vi "DSF Config File to Engine Config Cluster.vi"(8 "error in (no error)":errorcluster, 10 "engine offsets":u64[](array[numeric]), 11 "dsf configuration file path":path) -> (0 "error out":errorcluster, 3 "configuration cluster":T1)   [LabVIEW 2017, in "DSF.Engine.lvlib"]
uses:
  DSF.Engine.lvlib
  Shared/Typedefs/DSF.Shared.Refactor.Typedefs.Framework Configuration.Aggregate.JSON.ctl
  Shared/Typedefs/DSF.Shared.Refactor.Typedefs.Plugin Configuration.Aggregate.JSON.ctl
  Shared/Typedefs/DSF.Shared.Typedefs.Cycle Timing Factors.ctl
  Shared/Typedefs/DSF.Shared.Refactor.Typedefs.Transfer Group Configuration.Aggregate.JSON.ctl
  Shared/Typedefs/DSF.Shared.Refactor.Typedefs.JSON.Transfer Configuration.ctl
  Shared/Typedefs/DSF.Shared.Refactor.Typedefs.JSON.Channel Array Configuration.ctl
  Shared/Typedefs/DSF.Shared.Typedefs.Settings.Configuration.ctl
  DSF Configuration API/1.0.0/Public/Read All Item IDs/Read All Plugin IDs.vi
  DSF Configuration API/1.0.0/Public/Read Item/Read Plugin.vi
  DSF Configuration API/1.0.0/Public/Read Item/Read Settings.vi
  DSF Configuration API/1.0.0/Public/Read Item/Read Group.vi
  DSF Configuration API/1.0.0/Public/Read Item/Read Transfer.vi
  DSF Configuration API/1.0.0/Public/Read Item/Read Channel.vi
  DSF Configuration API/1.0.0/DSF Configuration API.lvlib
  DSF.Shared.lvlib
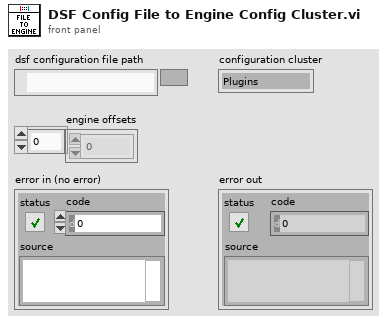
[diagram p1: front panel]
types:
  T1 = typedef "DSF.Shared.lvlib/DSF.Shared.Refactor.Typedefs.Framework Configuration.Aggregate.JSON.ctl" = cluster{"Plugins":T2[]}
  T2 = typedef "DSF.Shared.lvlib/DSF.Shared.Refactor.Typedefs.Plugin Configuration.Aggregate.JSON.ctl" = cluster{"name":string, "class":string, "cycle timing":T3, "Transfer Groups":T4[], "settings":T7[]}
  T3 = typedef "DSF.Shared.lvlib/DSF.Shared.Typedefs.Cycle Timing Factors.ctl" = cluster{"Priority":u64, "Decimation":u64, "Offset":u64}
  T4 = typedef "DSF.Shared.lvlib/DSF.Shared.Refactor.Typedefs.Transfer Group Configuration.Aggregate.JSON.ctl" = cluster{"name":string, "direction":u8, "cycle timing":T3, "Transfers":T5[], "settings":T7[]}
  T5 = typedef "DSF.Shared.lvlib/DSF.Shared.Refactor.Typedefs.JSON.Transfer Configuration.ctl" = cluster{"name":string, "byte order":u8, "channel configurations":T6[], "settings":T7[]}
  T6 = typedef "DSF.Shared.lvlib/DSF.Shared.Refactor.Typedefs.JSON.Channel Array Configuration.ctl" = cluster{"name":string, "data type":u8, "count":u64, "buffer offset":u64, "engine offset":u64, "settings":T7[]}
  T7 = typedef "DSF.Shared.lvlib/DSF.Shared.Typedefs.Settings.Configuration.ctl" = cluster{"key":string, "value":string}
  T8 = typedef "DSF Configuration API.lvlib/DSF Config Data RefNum.ctl" = refnum<k1>
  T9 = typedef "DSF Configuration API.lvlib/DSF Plugin Info.ctl" = cluster{"type":string, "timing":T10, "group ids":string[], "settings id":string}
  T10 = typedef "DSF Configuration API.lvlib/DSF Timing Info.ctl" = cluster{"priority":i32, "decimation":i32, "offset":i32}
  T11 = typedef "DSF Configuration API.lvlib/DSF Settings Info.ctl" = cluster{"key":string, "value":string}[]
  T12 = typedef "DSF Configuration API.lvlib/DSF Group Info.ctl" = cluster{"direction":T13, "timing":T10, "transfer ids":string[], "settings id":string}
  T13 = typedef "DSF Configuration API.lvlib/DSF Direction.ctl" = enum8{"Tx", "Rx"}
  T14 = typedef "DSF Configuration API.lvlib/DSF Transfer Info.ctl" = cluster{"byte order":T15, "channel ids":string[], "settings id":string}
  T15 = typedef "DSF Configuration API.lvlib/DSF Byte Order.ctl" = enum8{"big-endian", "little-endian"}
  T16 = typedef "DSF Configuration API.lvlib/DSF Channel Info.ctl" = cluster{"count":i32, "offset":i32, "data type":T17, "resource path":string, "settings id":string}
  T17 = typedef "DSF Configuration API.lvlib/DSF Data Type.ctl" = enum8{"Bool", "SGL", "DBL", "I8", "I16", "I32", "I64", "U8", "U16", "U32", "U64"}
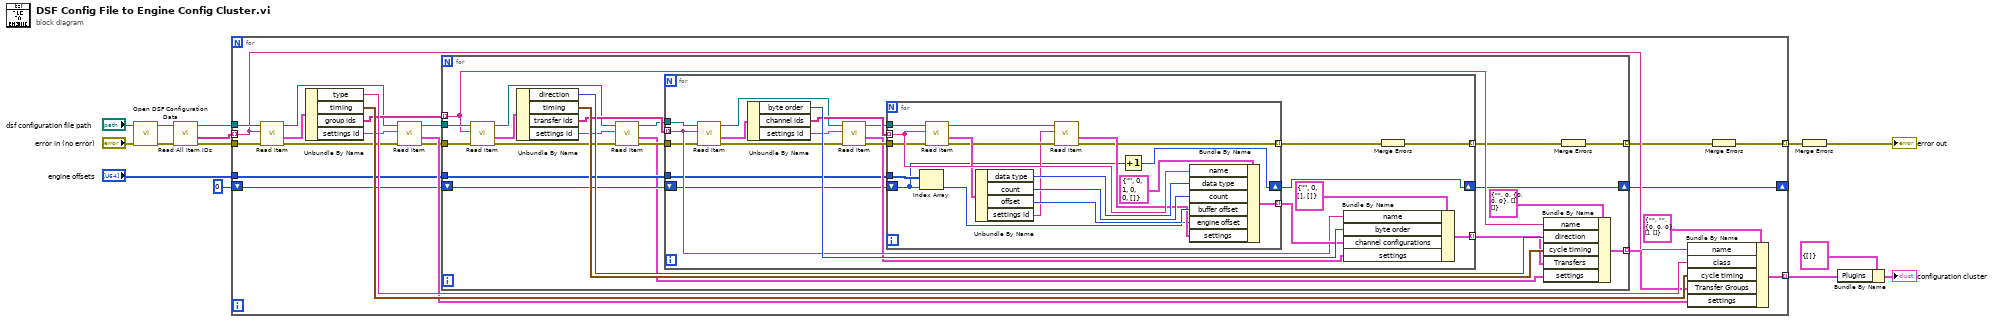
[diagram p0: block diagram]
diagram:
  n1 = call "Open DSF Configuration Data.vi"("error in (no error)"="error in (no error)", "dsf configuration file path"="dsf configuration file path") -> ("error out"=w11:errorcluster, "dsf refnum"=w12:T8)  [unwired: 6 in, 2 out]
  n2 = call-poly "Read All Item IDs.vi"("error in (no error)"=w11, "dsf refnum"=w12) -> ("error out"=w5:errorcluster, "Plugin IDs"=w9:string[], "dsf refnum out"=w8:T8)  [unwired: 7 in]
  n3 = for {
    tunnel: w9 -> [w27] mode=indexing
    tunnel: w8 -> [w34]
    tunnel: [w30] -> w7 mode=indexing
    tunnel: w5 -> [w21]
    tunnel: "engine offsets" -> [w19]
    shift-right: [w17] -> _
    shift-left: 0 -> [w18]
    tunnel: [w15] -> w2 mode=indexing
    n4 = call-poly "Read Item.vi"("error in (no error)"=w21, "Plugin ID"=w27, "dsf refnum"=w34) -> ("error out"=w22:errorcluster, "value"=w33:T9, "dsf refnum out"=w26:T8)  [unwired: 5 in, 1 out]
    n5 = Unbundle By Name(w33) -> ("type"=w32:string, "timing"=w31:T10, "group ids"=w29:string[], "settings id"=w24:string)
    n6 = call-poly "Read Item.vi"("error in (no error)"=w22, "Settings ID"=w24, "dsf refnum"=w26) -> ("error out"=w20:errorcluster, "value"=w23:T11, "dsf refnum out"=w25:T8)  [unwired: 5 in, 1 out]
    n7 = for {
      tunnel: w25 -> [w56]
      tunnel: w29 -> [w53] mode=indexing
      tunnel: [w50] -> w28 mode=indexing
      tunnel: w20 -> [w47]
      tunnel: w19 -> [w41]
      shift-right: [w39] -> w17
      shift-left: w18 -> [w40]
      tunnel: [w36] -> w16 mode=indexing
      n8 = call-poly "Read Item.vi"("error in (no error)"=w47, "Group ID"=w53, "dsf refnum"=w56) -> ("error out"=w43:errorcluster, "value"=w54:T12, "dsf refnum out"=w46:T8)  [unwired: 5 in, 1 out]
      n9 = Unbundle By Name(w54) -> ("direction"=w52:T13, "timing"=w51:T10, "transfer ids"=w49:string[], "settings id"=w44:string)
      n10 = call-poly "Read Item.vi"("error in (no error)"=w43, "Settings ID"=w44, "dsf refnum"=w46) -> ("error out"=w42:errorcluster, "value"=w38:T11, "dsf refnum out"=w45:T8)  [unwired: 5 in, 1 out]
      n11 = for {
        tunnel: w49 -> [w68] mode=indexing
        tunnel: w45 -> [w76]
        tunnel: [w72] -> w48 mode=indexing
        tunnel: w42 -> [w67]
        tunnel: w41 -> [w61]
        shift-right: [w59] -> w39
        shift-left: w40 -> [w60]
        tunnel: [w57] -> w37 mode=indexing
        n12 = call-poly "Read Item.vi"("error in (no error)"=w67, "Transfer ID"=w68, "dsf refnum"=w76) -> ("error out"=w65:errorcluster, "value"=w75:T14, "dsf refnum out"=w69:T8)  [unwired: 5 in, 1 out]
        n13 = Unbundle By Name(w75) -> ("byte order"=w73:T15, "channel ids"=w70:string[], "settings id"=w64:string)
        n14 = call-poly "Read Item.vi"("error in (no error)"=w65, "Settings ID"=w64, "dsf refnum"=w69) -> ("error out"=w63:errorcluster, "value"=w62:T11, "dsf refnum out"=w66:T8)  [unwired: 5 in, 1 out]
        n15 = for {
          tunnel: [w93] -> w71 mode=indexing
          tunnel: w70 -> [w91] mode=indexing
          tunnel: w66 -> [w92]
          tunnel: w63 -> [w86]
          tunnel: w61 -> [w81]
          shift-right: [w79] -> w59
          shift-left: w60 -> [w80]
          tunnel: [w77] -> w58 mode=indexing
          n16 = Index Array(array=w81, index=w80) -> (element=w78:u64)
          n17 = call-poly "Read Item.vi"("error in (no error)"=w86, "Channel ID"=w91, "dsf refnum"=w92) -> ("error out"=w84:errorcluster, "value"=w90:T16, "dsf refnum out"=w85:T8)  [unwired: 5 in, 1 out]
          n18 = Unbundle By Name(w90) -> ("data type"=w89:T17, "count"=w88:i32, "offset"=w87:i32, "settings id"=w83:string)
          n19 = call-poly "Read Item.vi"("error in (no error)"=w84, "Settings ID"=w83, "dsf refnum"=w85) -> ("error out"=w77:errorcluster, "value"=w82:T11)  [unwired: 5 in, 2 out]
          n20 = Increment(x=w80) -> (x+1=w79:i32)
          n21 = Bundle By Name(cluster=T6 {"name"="", "data type"=0, "count"=1, "buffer offset"=0, "engine offset"=0, "settings"=[]} ("channel configurations"), "name"=w91, "data type"=w89, "count"=w88, "buffer offset"=w87, "engine offset"=w78, "settings"=w82) -> (w93:T6)
        }
        n22 = Bundle By Name(cluster=T5 {"name"="", "byte order"=0, "channel configurations"=[], "settings"=[]} ("Transfers"), "name"=w68, "byte order"=w73, "channel configurations"=w71, "settings"=w62) -> (w72:T5)
        n23 = Merge Errors(w58) -> (w57:errorcluster)
      }
      n24 = Bundle By Name(cluster=T4 {"name"="", "direction"=0, "cycle timing"={"Priority"=0, "Decimation"=0, "Offset"=0}, "Transfers"=[], "settings"=[]} ("Transfer Group Configuration"), "name"=w53, "direction"=w52, "cycle timing"=w51, "Transfers"=w48, "settings"=w38) -> (w50:T4)
      n25 = Merge Errors(w37) -> (w36:errorcluster)
    }
    n26 = Bundle By Name(cluster=T2 {"name"="", "class"="", "cycle timing"={"Priority"=0, "Decimation"=0, "Offset"=0}, "Transfer Groups"=[], "settings"=[]} ("Plugin Configuration"), "name"=w27, "class"=w32, "cycle timing"=w31, "Transfer Groups"=w28, "settings"=w23) -> (w30:T2)
    n27 = Merge Errors(w16) -> (w15:errorcluster)
  }
  n28 = Merge Errors(w2) -> (→"error out":errorcluster)
  n29 = Bundle By Name(cluster=T1 {"Plugins"=[]} ("Framework Config (JSON)"), "Plugins"=w7) -> (→"configuration cluster":T1)
